vi "Properties Lookup.vi"() -> ()   [LabVIEW 2024, in "Protection and Counter Support Shared.lvlib"]
doc: "Use this Global VI to access the GUIDs assigned to the page resources of the Custom Device."
uses:
  Protection and Counter Support Shared.lvlib
panel:
  in  "Invalid Count Name":string="Invalid Count"
  in  "Value Name":string="Value"
  in  "Override Value Name":string="Override Value"
  in  "Override Name":string="Override"
  in  "Counter Value":string="Rolling Counter"
  in  "Protection Signals":string="Protection Signals"
  in  "Protection Type":string="Protection Type"
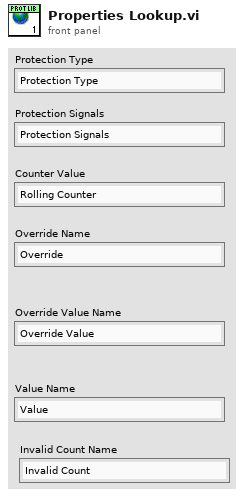
[diagram p1: front panel]
diagram:
